vi "VisionBinCoordinates.vi"(5 "Distance to Bin":dbl=nan, 6 "error in":errorcluster, 7 "Minimum Ratio":dbl=0.15, 8 "socket in":refnum<class "zmq_socket.lvclass">) -> (0 "x Coordinate of Bin":dbl, 1 "y Coordinate of Bin":dbl, 2 "bin angle":dbl, 3 "bin ratio":dbl, 4 "no bin detected":bool)   [LabVIEW 2015]
uses:
  <vilib>/Analysis/Matrix/Datatypes/RealMatrix.ctl
  labview-zmq/zmq_socket.lvclass
  labview-zmq/socket_type.ctl
  labview-zmq/socket_options.ctl
  <vilib>/Analysis/Matrix/Numeric/Conversions/Array To Matrix - RA2.vi
  <vilib>/Analysis/Matrix/NI_Matrix.lvlib
  labview-zmq/zmq_context.lvclass
  labview-zmq/zeromq.lvlib
  <vilib>/Rock Robotics/Network Tables/NT Read Number.vi
panel:
  in  "y":bool
  out "Real Matrix":T1
  out "data":string
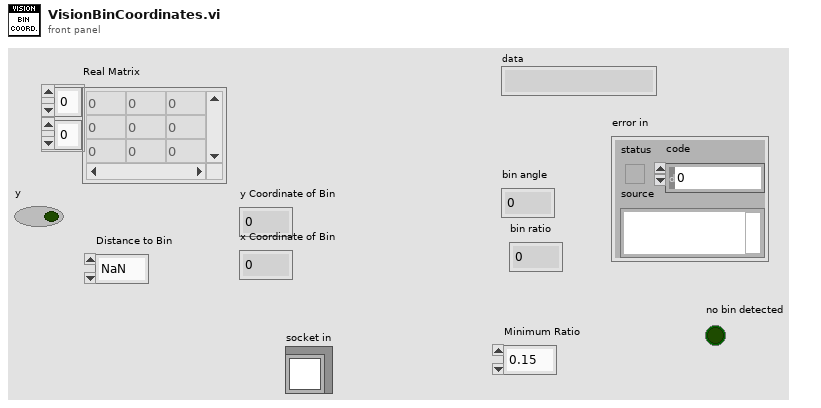
[diagram p1: front panel]
types:
  T1 = typedef "NI_Matrix.lvlib/RealMatrix.ctl" = dbl[][]
  T2 = typedef "zeromq.lvlib/socket_options.ctl" = enum8{"NONE", "ZMQ_HWM", "<2>", "ZMQ_SWAP", "ZMQ_AFFINITY", "ZMQ_IDENTITY", "ZMQ_SUBSCRIBE", "ZMQ_UNSUBSCRIBE", "ZMQ_RATE", "ZMQ_RECOVERY_IVL", "ZMQ_MCAST_LOOP", "ZMQ_SNDBUF", "ZMQ_RCVBUF", "ZMQ_RCVMORE", "ZMQ_FD", "ZMQ_EVENTS", "ZMQ_TYPE", "ZMQ_LINGER", "ZMQ_RECONNECT_IVL", "ZMQ_BACKLOG", "ZMQ_RECOVERY_IVL_MSEC", "ZMQ_RECONNECT_IVL_MAX", "ZMQ_MAXMSGSIZE", "ZMQ_SNDHWM", "ZMQ_RCVHWM", "ZMQ_MULTICAST_HOPS", "<26>", "ZMQ_RCVTIMEO", "ZMQ_SNDTIMEO", "<29>", "<30>", "ZMQ_IPV4ONLY", "ZMQ_LAST_ENDPOINT", "ZMQ_ROUTER_MANDATORY", "ZMQ_TCP_KEEPALIVE", "ZMQ_TCP_KEEPALIVE_CNT", "ZMQ_TCP_KEEPALIVE_IDLE", "ZMQ_TCP_KEEPALIVE_INTVL", "ZMQ_TCP_ACCEPT_FILTER", "ZMQ_DELAY_ATTACH_ON_CONNECT", "ZMQ_XPUB_VERBOSE"}
  T3 = typedef "zeromq.lvlib/socket_type.ctl" = enum8{"ZMQ_PAIR", "ZMQ_PUB", "ZMQ_SUB", "ZMQ_REQ", "ZMQ_REP", "ZMQ_DEALER", "ZMQ_ROUTER", "ZMQ_PULL", "ZMQ_PUSH", "ZMQ_XPUB", "ZMQ_XSUB"}
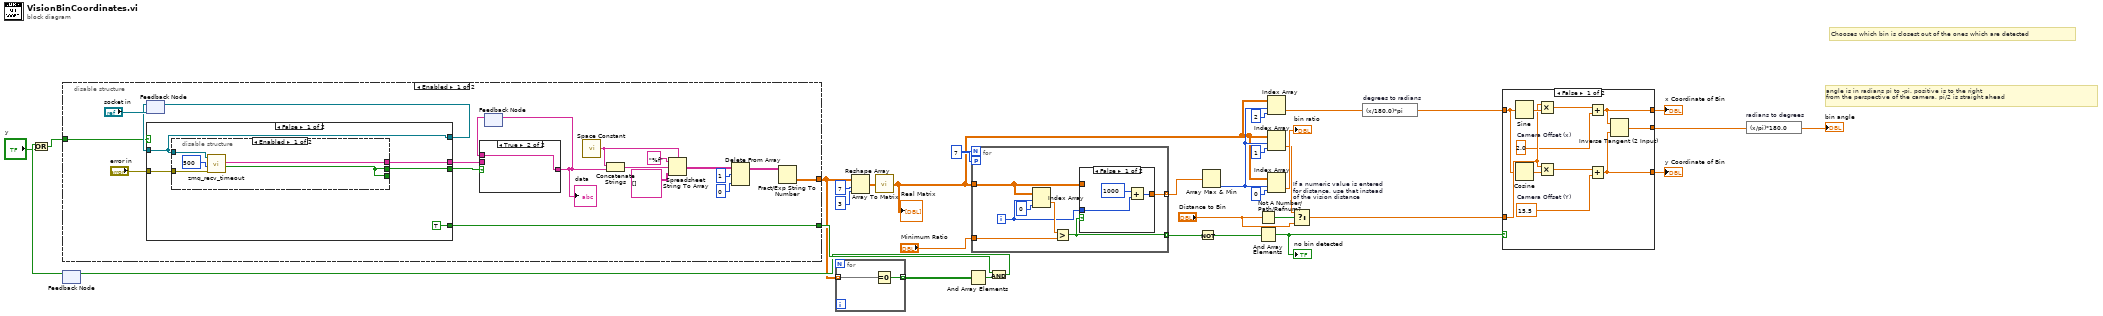
[diagram p0: block diagram]
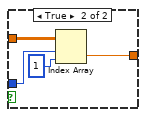
[diagram p2: hidden frame]
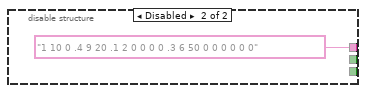
[diagram p3: hidden frame]
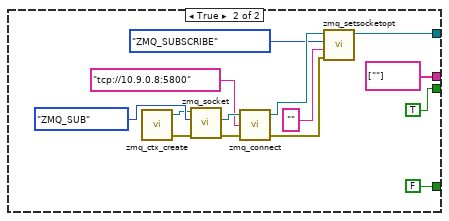
[diagram p4: hidden frame]
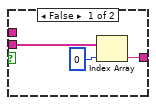
[diagram p5: hidden frame]
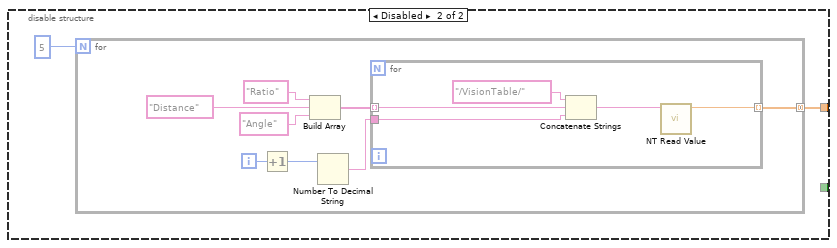
[diagram p6: hidden frame]
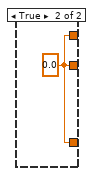
[diagram p7: hidden frame]
diagram:
  w25 = 7
  # "angle is in radians pi to -pi. positive is to the right \nfrom the perspective of the camera, pi/2 is straight ahead"
  # "Chooses which bin is closest out of the ones which are detected"
  n1 = feedback #1() -> (w3:bool)  [unwired: 1 in]
  n2 = Or(x=w3, y="y") -> (x .or. y?=w1:bool)
  n3 = disable-structure shown="Enabled" {
    disable-tunnel: [w46 w83] -> w4
    disable-tunnel: w1 -> [w34 _]
    disable-tunnel: [w35 _] -> w6
    frame Enabled {
      n4 = feedback #2("socket in") -> (w37:refnum<class "zmq_socket.lvclass">)
      n5 = case shown="False" w34 {
        tunnel: [w57 string[] [""] ("parts")] -> w41
        tunnel: [w56 TRUE ("timeout?")] -> w40
        tunnel: w37 -> [w55 _]
        tunnel: [w55 w65] -> w39
        tunnel: "error in" -> [w54 _]
        tunnel: [TRUE FALSE] -> w35
        frame False {
          n6 = disable-structure shown="Enabled" {
            disable-tunnel: [w62 "1 10 0 .4 9 20 .1 2 0 0 0 0 .3 6 50 0 0 0 0 0 0"] -> w57
            disable-tunnel: [w60 _] -> w56
            disable-tunnel: w54 -> [w59 _]
            disable-tunnel: [w60 _] -> _
            disable-tunnel: w55 -> [w58 _]
            frame Enabled {
              n7 = call "zmq_recv_timeout.vi"("error in"=w59, "timeout (ms)"=u32 500, "socket in"=w58) -> ("timeout?"=w60:bool, "parts"=w62:string[])  [unwired: 1 in, 2 out]
            }
            frame Disabled {
            }
          }
        }
        frame True {
          n8 = call "zmq_ctx_create.vi"() -> ("error out"=w73:errorcluster, "context out"=w76:refnum<class "zmq_context.lvclass">)  [unwired: 4 in]
          n9 = call "zmq_socket.vi"("error in"=w73, "socket type"=socket_type."ZMQ_SUB", "context in"=w76) -> ("error out"=w70:errorcluster, "socket out"=w75:refnum<class "zmq_socket.lvclass">)  [unwired: 2 in, 1 out]
          n10 = call "zmq_connect.vi"("error in"=w70, "endpoint"="tcp://10.9.0.8:5800" ("Endpoint"), "socket in"=w75) -> ("error out"=w71:errorcluster, "socket out"=w72:refnum<class "zmq_socket.lvclass">)  [unwired: 1 in]
          n11 = call "zmq_setsocketopt.vi"("error in"=w71, "value"="", "option"=socket_options."ZMQ_SUBSCRIBE", "socket in"=w72) -> ("socket out"=w65:refnum<class "zmq_socket.lvclass">)  [unwired: 2 in, 1 out]
        }
      }
      n12 = feedback-in #2(w39) -> ()
      n13 = feedback #3() -> (w42:string)  [unwired: 1 in]
      n14 = case shown="True" w40 {
        tunnel: w41 -> [w80 _]
        tunnel: [w78 w81] -> w43
        tunnel: w42 -> [_ w81]
        frame False {
          n15 = Index Array(array=w80, index=0) -> (element=w78:string)
        }
        frame True {
        }
      }
      "data" <- w43
      n16 = feedback-in #3(w43) -> ()
      n17 = call <vilib>:"Space Constant.vi"() -> ("String"=w44:string)
      n18 = Concatenate Strings(w44, w43) -> (w45:string)
      n19 = Spreadsheet String To Array(delimiter (Tab)=w44, format string="%f", spreadsheet string=w45, array type (2D Dbl)=string[][] [] ("Array")) -> (array=w47:string[][])
      n20 = Delete From Array(array=w47, length=1, index (col)=0 ("disabled index (col)")) -> (array with subset deleted=w48:string[][])  [unwired: 1 in, 1 out]
      n21 = Fract/Exp String To Number(string=w48) -> (number=w46:dbl[][])  [unwired: 4 out]
    }
    frame Disabled {
      n22 = for {
        N: 5 -> [_]
        tunnel: [w91] -> w83 mode=concatenating
        i -> [w86]
        n23 = Increment(x=w86) -> (x+1=w85:i32)
        n24 = Build Array("Ratio" ("element"), "Distance" ("element"), "Angle") -> (w87:string[])
        n25 = Number To Decimal String(number=w85) -> (decimal integer string=w84:string)  [unwired: 1 in]
        n26 = for {
          tunnel: [w95] -> w91 mode=indexing
          tunnel: w87 -> [w94] mode=indexing
          tunnel: w84 -> [w92]
          n27 = Concatenate Strings("/VisionTable/" ("string"), w94, w92) -> (w96:string)
          n28 = call-poly <vilib>:"NT Read Value.vi"("Name"=w96) -> ("Numeric"=w95:dbl)  [unwired: 9 in, 1 out]
        }
      }
    }
  }
  n29 = for {
    tunnel: w4 -> [w98] mode=indexing
    tunnel: [w97] -> w8 mode=indexing
    n30 = Equal To 0?(x=w98) -> (x = 0?=w97:bool[])
  }
  n31 = Reshape Array(w4, 7 ("dimension size"), 3 ("dimension size")) -> (w26:dbl[][])
  n32 = call-poly <vilib>:"Array To Matrix.vi"("Real 2D Array"=w26) -> ("Real Matrix"=w12:T1)
  "Real Matrix" <- w12
  n33 = And Array Elements(Boolean array=w8) -> (logical AND=w7:bool)
  n34 = for {
    N: w25 -> [_]
    workers-P: w25 -> [_]
    tunnel: w12 -> [w102]
    tunnel: "Minimum Ratio" -> [w104]
    tunnel: [w101] -> w23 mode=indexing
    tunnel: [w99] -> w14 mode=indexing
    i -> [w100]
    n35 = Index Array(array=w102, index (row)=w100, index (col)=0) -> (element=w105:dbl)
    n36 = Greater?(x=w105, y=w104) -> (0:w99:bool)
    n37 = case shown="False" w99 {
      tunnel: w100 -> [w106 w112]
      tunnel: w102 -> [_ w110]
      tunnel: [w107 w109] -> w101
      frame False {
        n38 = Add(x=1000, y=w106) -> (x+y=w107:i32)
      }
      frame True {
        n39 = Index Array(array=w110, index (row)=w112, index (col)=1) -> (element=w109:dbl)
      }
    }
  }
  n40 = And(x=w6, y=w7) -> (x .and. y?=w5:bool)
  n41 = feedback-in #1(w5) -> ()
  n42 = Not(x=w14) -> (.not. x?=w15:bool[])
  n43 = Array Max & Min(array=w23) -> (min index (indices)=w16:i32)  [unwired: 3 out]
  n44 = Not A Number/Path/Refnum?(number/path/refnum="Distance to Bin") -> (NaN/Path/Refnum?=w33:bool)
  n45 = And Array Elements(Boolean array=w15) -> (logical AND=w13:bool)
  "no bin detected" <- w13
  n46 = Index Array(array=w12, index (row)=w16, index (col)=2) -> (element=w11:dbl)
  n47 = Index Array(array=w12, index (row)=w16, index (col)=1) -> (element=w17:dbl)
  n48 = Index Array(array=w12, index (row)=w16, index (col)=0) -> (element=→"bin ratio":dbl)
  n49 = Select "If a numeric value is entered\nfor distance, use that instead\nof the vision distance"(t=w17, s=w33, f="Distance to Bin") -> (s? t:f=w19:dbl)
  n50 = expression code="(x/180.0)*pi" "degrees to radians"(w11) -> (w29:dbl)
  n51 = case shown="False" w13 {
    tunnel: w29 -> [w119 _]
    tunnel: w19 -> [w121 _]
    tunnel: [w116 w124] -> w31
    tunnel: [w115 w124] -> w30
    tunnel: [w117 w124] -> w10
    frame False {
      w113 = 15.5  # Camera Offset (Y)
      w114 = 2.0  # Camera Offset (x)
      n52 = Sine(x=w119) -> (sin(x)=w122:dbl)
      n53 = Cosine(x=w119) -> (cos(x)=w123:dbl)
      n54 = Multiply(x=w121, y=w122) -> (x*y=w120:dbl)
      n55 = Multiply(x=w121, y=w123) -> (x*y=w118:dbl)
      n56 = Add(x=w120, y=w114) -> (x+y=w115:dbl)
      n57 = Add(x=w118, y=w113) -> (x+y=w116:dbl)
      n58 = Inverse Tangent (2 Input)(1:w116, 2:w115) -> (0:w117:dbl)
    }
    frame True {
      w124 = 0.0
    }
  }
  "y Coordinate of Bin" <- w31
  "x Coordinate of Bin" <- w30
  n59 = expression code="(x/pi)*180.0" "radians to degrees"(w10) -> (→"bin angle":dbl)
